vi "Update Open Dir.vi"(8 "error in (no error)":errorcluster, 9 "Size to Add":i64, 10 "open dir":refnum<class "dir.lvclass">, 11 "dir in":refnum<class "dir.lvclass">) -> (0 "error out":errorcluster, 3 "dir out":refnum<class "dir.lvclass">)   [LabVIEW 2021, in "d7.lvlib" / "dir.lvclass"]
uses:
  dir.lvclass
  C:/Projects/lv2021-advent-of-code-2022/d7/INode/INode.lvclass
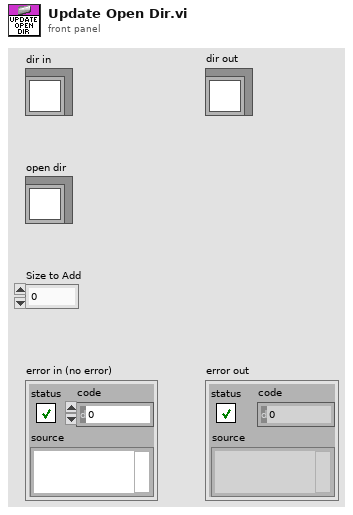
[diagram p1: front panel]
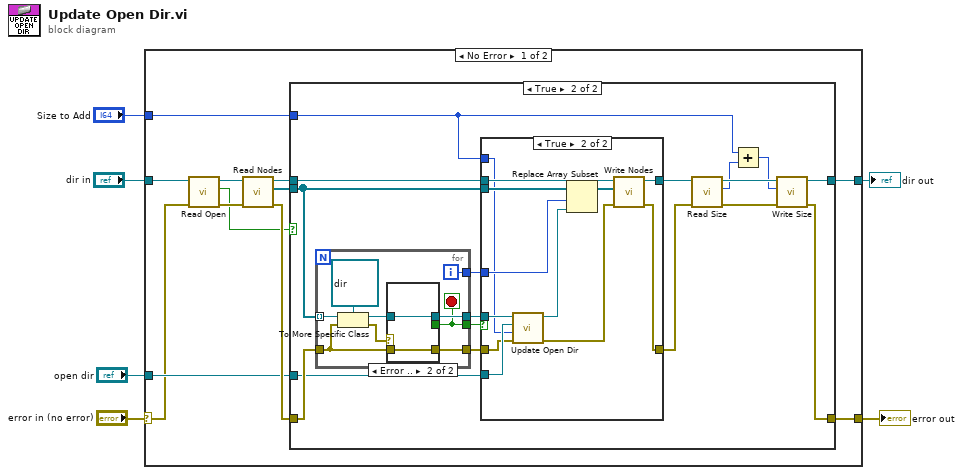
[diagram p0: block diagram]
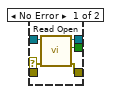
[diagram p4: hidden frame]
diagram:
  n1 = case shown="No Error" "error in (no error)" {
    selector: "error in (no error)" -> [w10 w68]
    tunnel: "dir in" -> [w11 w69]
    tunnel: "open dir" -> [w17 _]
    tunnel: [w15 w69] -> w3
    tunnel: [w13 w68] -> w2
    tunnel: "Size to Add" -> [w7 _]
    frame No Error {
      n2 = call-dynamic "Read Open.vi"("error in (no error)"=w10, "dir in"=w11) -> ("error out"=w9:errorcluster, "Open"=w8:bool, "dir out"=w12:refnum<class "dir.lvclass">)  [unwired: 7 in]
      n3 = call-dynamic "Read Nodes.vi"("error in (no error)"=w9, "dir in"=w12) -> ("error out"=w18:errorcluster, "Nodes"=w14:refnum<class "INode.lvclass">[], "dir out"=w16:refnum<class "dir.lvclass">)  [unwired: 7 in]
      n4 = case shown="True" w8 {
        tunnel: w18 -> [w19 w37]
        tunnel: w17 -> [w20 w36]
        tunnel: w16 -> [_ w35]
        tunnel: [w20 w26] -> w15
        tunnel: w14 -> [_ w32]
        tunnel: [w19 w25] -> w13
        tunnel: w7 -> [_ w21]
        frame False {
        }
        frame True {
          n5 = for {
            tunnel: [w57] -> w34
            tunnel: w32 -> [w52] mode=indexing
            tunnel: w37 -> [w53]
            tunnel: [w56] -> w33
            tunnel: [w55] -> w30
            tunnel: [w54] -> w31
            i -> [w54]
            stop <- w55 stop-if-true
            n6 = To More Specific Class(target class=refnum<class "dir.lvclass"> refnum, reference=w52, error in=w53) -> (specific class reference=w59:refnum<class "dir.lvclass">, error out=w58:errorcluster)
            n7 = case shown="Error .." w58 {
              selector: w58 -> [w64 _]
              tunnel: w59 -> [w65 w66]
              tunnel: [w63 w66] -> w57
              tunnel: [w62 w67] -> w56
              tunnel: [w61 _] -> w55
              tunnel: w53 -> [_ w67]
              frame No Error {
                n8 = call-dynamic "Read Open.vi"("error in (no error)"=w64, "dir in"=w65) -> ("error out"=w62:errorcluster, "Open"=w61:bool, "dir out"=w63:refnum<class "dir.lvclass">)  [unwired: 7 in]
              }
              frame Error {
              }
            }
          }
          n9 = case shown="True" w30 {
            tunnel: w36 -> [w39 w51]
            tunnel: w35 -> [_ w50]
            tunnel: [w39 w49] -> w27
            tunnel: [w38 w48] -> w29
            tunnel: w34 -> [_ w47]
            tunnel: w33 -> [w38 w46]
            tunnel: w32 -> [_ w42]
            tunnel: w31 -> [_ w41]
            tunnel: w21 -> [_ w40]
            frame False {
            }
            frame True {
              n10 = call "Update Open Dir.vi"("error in (no error)"=w46, "Size to Add"=w40, "open dir"=w51, "dir in"=w47) -> ("error out"=w43:errorcluster, "dir out"=w44:refnum<class "dir.lvclass">)  [unwired: 6 in]
              n11 = Replace Array Subset(array=w42, new element=w44, index=w41) -> (w45:refnum<class "INode.lvclass">[])
              n12 = call-dynamic "Write Nodes.vi"("error in (no error)"=w43, "Nodes"=w45, "dir in"=w50) -> ("error out"=w48:errorcluster, "dir out"=w49:refnum<class "dir.lvclass">)  [unwired: 7 in]
            }
          }
          n13 = call-dynamic "Read Size.vi"("error in (no error)"=w29, "file in"=w27) -> ("error out"=w22:errorcluster, "Size"=w24:i64, "file out"=w28:refnum<class "dir.lvclass">)  [unwired: 7 in]
          n14 = Add(x=w21, y=w24) -> (x+y=w23:i64)
          n15 = call-dynamic "Write Size.vi"("error in (no error)"=w22, "Size"=w23, "file in"=w28) -> ("error out"=w25:errorcluster, "file out"=w26:refnum<class "dir.lvclass">)  [unwired: 7 in]
        }
      }
    }
    frame Error {
    }
  }
  "error out" <- w2
  "dir out" <- w3
